vi "ITR LP order 3.vi"(7 "input":dbl format="%.2f", 13 "corner period (steps)":dbl(slide)=10.237739663395852 scale=1.0..1000.0) -> (8 "output":dbl format="%.2f")   [LabVIEW 2016]
doc: "Modular ITR third order low pass filter with internal shift registers.\n\nAlexis Lopez\nP350\nCSUSB Physics"
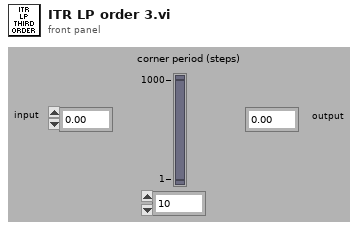
[diagram p1: front panel]
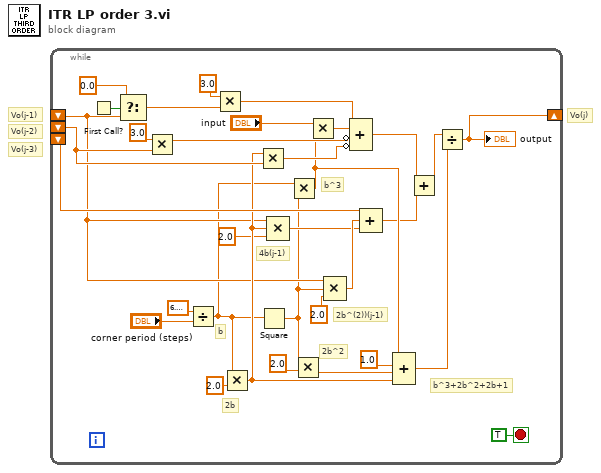
[diagram p0: block diagram]
diagram:
  # "Vo(j-3)"
  # "Vo(j-2)"
  # "Vo(j-1)"
  # "Vo(j)"
  n1 = while {
    shift-left: _ -> [w11]
    shift-right: [w27] -> _
    shift-left: _ -> [w18]
    shift-left: _ -> [w16]
    stop <- TRUE stop-if-true
    # "b^3"
    # "2b^(2))(j-1)"
    # "2b^2"
    # "4b(j-1)"
    # "2b"
    # "b^3+2b^2+2b+1"
    # "b"
    n2 = First Call?() -> (First Call?: T/F=w24:bool)
    n3 = Select(t=0.0, s=w24, f=w11) -> (s? t:f=w22:dbl)
    n4 = Multiply(x=3.0, y=w18) -> (x*y=w19:dbl)
    n5 = Divide(x=6.283185307179586, y="corner period (steps)") -> (x/y=w8:dbl)
    n6 = Multiply(x=3.0, y=w22) -> (x*y=w23:dbl)
    n7 = Multiply(x=w8, y=2.0) -> (x*y=w14:dbl)
    n8 = Multiply(x=w14, y=w18) -> (x*y=w20:dbl)
    n9 = Square(x=w8) -> (x^2=w6:dbl)
    n10 = Compound Arithmetic op=MULTIPLY(w11, w14, 2.0) -> (w9:dbl)
    n11 = Multiply(x=w8, y=w6) -> (x*y=w4:dbl)
    n12 = Multiply(x=w6, y=2.0) -> (x*y=w7:dbl)
    n13 = Multiply(x="input", y=w4) -> (x*y=w26:dbl)
    n14 = Compound Arithmetic op=MULTIPLY(w11, w6, 2.0) -> (w10:dbl)
    n15 = Compound Arithmetic op=ADD(w23, w26, invert w19, invert w20) -> (w3:dbl)
    n16 = Compound Arithmetic op=ADD(w16, w10, w9) -> (w2:dbl)
    n17 = Compound Arithmetic op=ADD(w4, 1.0, w7, w14) -> (w28:dbl)
    n18 = Add(x=w3, y=w2) -> (x+y=w1:dbl)
    n19 = Divide(x=w1, y=w28) -> (x/y=w27:dbl)
    "output" <- w27
  }
